vi "PreCompileMetaSeq.vi"(6 "steps":i32, 8 "error in (no error)":errorcluster, 10 "Compiler Settings":T1={"Python Path"=path "", "Main File"="", "Meta File"="", "Aux File"="", "Pre File"="metascript.txt"}, 11 "queue in":refnum<queue>) -> (0 "error out":errorcluster, 3 "calib":bool)   [LabVIEW 2019]
uses:
  PulseCompiler/CompilerSettings.ctl
  Controller/PulseControl.ctl
  Params.ctl
  controls/GlobalExp.vi
  Global.lvlib
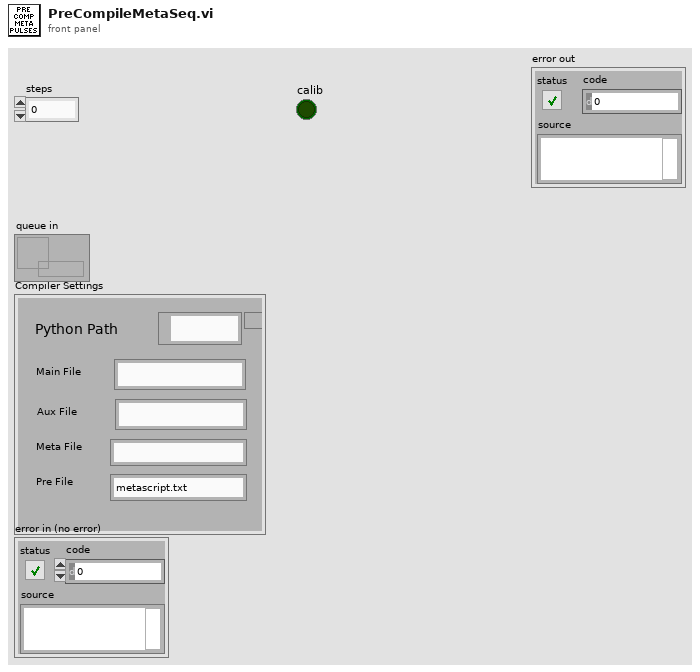
[diagram p1: front panel]
types:
  T1 = typedef "CompilerSettings.ctl" = cluster{"Python Path":path, "Main File":string, "Meta File":string, "Aux File":string, "Pre File":string}
  T2 = typedef "PulseControl.ctl" = cluster{"FPGA Code":cluster{"Times":u32[], "Pulses":u64[], "Counts":u8[], "Triggers":u8[], "AOs":u8[], "# of runs":i32, "Line trig?":bool, "time photons?":bool}, "AWG pulses array":variant[], "Params":T3}
  T3 = typedef "Params.ctl" = cluster{"steps":i16, "runs":i16, "comment":string, "mathematica":string, "calib":i8, "logmsg":string, "ndets":i16}
  T4 = typedef "MasterExpControl.ctl" = cluster{"Main Steps":dbl, "Main Runs":dbl, "ExpStatus":enum16{"Innit", "Stop", "Idle", "MainRunning", "AuxRunning"}, "Main Current Step":dbl, "ExpNum":dbl, "NewData":bool, "date":string, "command":string, "Stop":bool, "Pause":bool, "Mathematica":string, "Main/Meta":bool, "UpdateMath":bool, "Camera":bool, "MetaExpOver":bool, "NextMetaExp":bool}
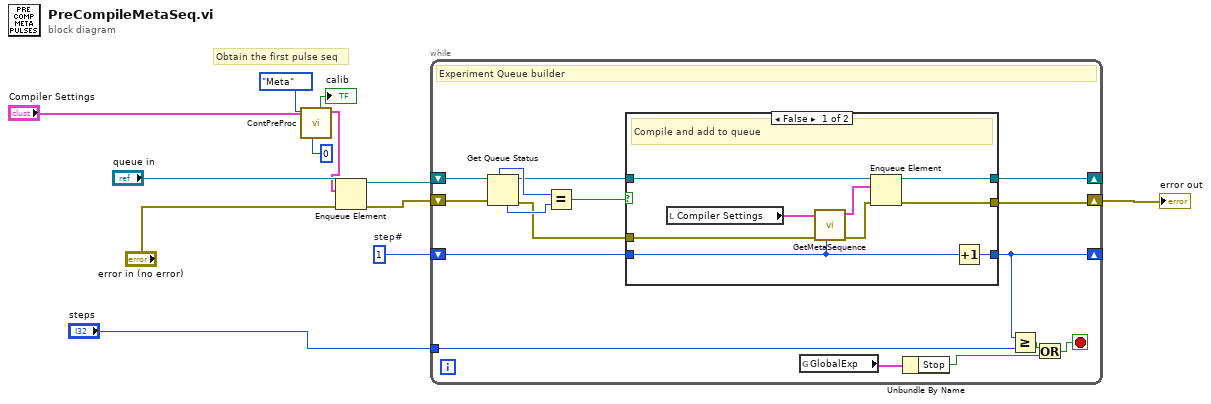
[diagram p0: block diagram]
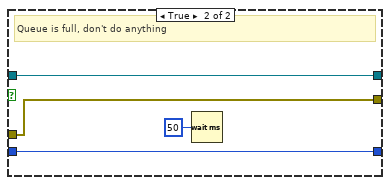
[diagram p2: hidden frame]
diagram:
  w5 = 1  # step#
  # "Obtain the first pulse seq"
  n1 = call "ContPreProc.vi"("step num"=0, "Compiler Settings"="Compiler Settings", "Enum"=enum16{"Meta", "Aux", "Main"}."Meta") -> ("Main pulse seq"=w7:T2, "calib"=→"calib":bool)  [unwired: 4 in, 3 out]
  n2 = Enqueue Element(queue="queue in", element=w7, error in (no error)="error in (no error)") -> (queue out=w9:refnum<queue>, error out=w10:errorcluster)  [unwired: 1 in, 1 out]
  n3 = while {
    shift-right: [w22] -> _
    shift-left: w5 -> [w24]
    tunnel: "steps" -> [w23]
    shift-right: [w20] -> _
    shift-left: w9 -> [w28]
    shift-right: [w17] -> w1
    shift-left: w10 -> [w19]
    stop <- w15 stop-if-true
    # "Experiment Queue builder"
    n4 = Get Queue Status(queue=w28, error in (no error)=w19) -> (queue out=w21:refnum<queue>, max queue size=w27:i32, error out=w18:errorcluster, # elements in queue=w26:i32)  [unwired: 1 in, 4 out]
    n5 = Equal?(x=w27, y=w26) -> (x = y?=w25:bool)
    n6 = case shown="False" w25 {
      tunnel: w24 -> [w36 w41]
      tunnel: [w37 w41] -> w22
      tunnel: w21 -> [w35 w40]
      tunnel: [w34 w40] -> w20
      tunnel: w18 -> [w32 w38]
      tunnel: [w30 w38] -> w17
      frame False {
        # "Compile and add to queue"
        n7 = local read "Compiler Settings"() -> (w29:T1)
        n8 = call "GetMetaSequence.vi"("Stepnum"=w36, "error in (no error)"=w32, "Compiler Settings"=w29) -> ("error out"=w31:errorcluster, "Main pulse"=w33:T2)  [unwired: 7 in]
        n9 = Enqueue Element(queue=w35, element=w33, error in (no error)=w31) -> (queue out=w34:refnum<queue>, error out=w30:errorcluster)  [unwired: 1 in, 1 out]
        n10 = Increment(x=w36) -> (x+1=w37:i32)
      }
      frame True {
        # "Queue is full, don't do anything"
        n11 = Wait (ms)(milliseconds to wait=u32 50) -> ()  [unwired: 1 out]
      }
    }
    n12 = global read "GlobalExp.vi" "GlobalExp"() -> (w14:T4)
    n13 = Unbundle By Name(w14) -> ("Stop"=w13:bool)
    n14 = Greater Or Equal?(x=w22, y=w23) -> (x >= y?=w16:bool)
    n15 = Or(x=w16, y=w13) -> (x .or. y?=w15:bool)
  }
  "error out" <- w1
